vi "LJM logger get file name.vi"(6 "Data File Extension":string="dat", 9 "Starting #":u32, 10 "Data File Prefix":string="data", 11 "Working Directory":path) -> (1 "Data File #":u32, 3 "Data File Path":path)   [LabVIEW 2026]
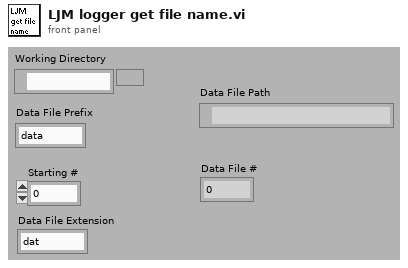
[diagram p1: front panel]
types:
  T1 = enum16{"open", "replace", "create", "open or create", "replace or create", "replace or create with confirmation"}
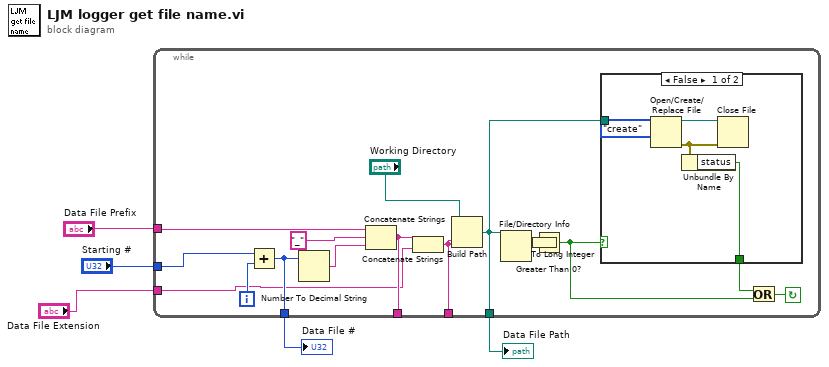
[diagram p0: block diagram]
diagram:
  n1 = while {
    tunnel: [w8] -> w2
    tunnel: "Starting #" -> [w10]
    tunnel: [w16] -> _
    tunnel: [w15] -> w4
    tunnel: [w17] -> _
    tunnel: "Data File Prefix" -> [w19]
    tunnel: "Data File Extension" -> [w7]
    i -> [w9]
    stop <- w14 continue-if-true
    n2 = Add(x=w10, y=w9) -> (x+y=w8:u32)
    n3 = Number To Decimal String(number=w8) -> (decimal integer string=w21:string)  [unwired: 1 in]
    n4 = Concatenate Strings(w19, "_" ("Substring"), w21) -> (w16:string)
    n5 = Concatenate Strings(w16, w7) -> (w17:string)
    n6 = Build Path(base path="Working Directory", name or relative path=w17) -> (appended path=w15:path)
    n7 = File/Directory Info(path=w15) -> (size=w6:i64)  [unwired: 1 in, 6 out]
    n8 = To Long Integer(number=w6) -> (32bit integer=w20:i32)
    n9 = Greater Than 0?(x=w20) -> (x > 0?=w11:bool)
    n10 = case shown="False" w11 {
      selector: w11 -> [_ w27]
      tunnel: w15 -> [w26 _]
      tunnel: [w24 w27] -> w13
      frame False {
        n11 = Open/Create/Replace File(file path (use dialog)=w26, operation (0:open)=T1."create") -> (refnum out=w23:refnum<file>, error out=w25:errorcluster)  [unwired: 4 in, 1 out]
        n12 = Unbundle By Name(w25) -> ("status"=w24:bool)
        n13 = Close File(refnum=w23, error in=w25) -> ()  [unwired: 2 out]
      }
      frame True {
      }
    }
    n14 = Or(x=w13, y=w11) -> (x .or. y?=w14:bool)
  }
  "Data File Path" <- w4
  "Data File #" <- w2
